vi "Init Actor Core.vi"(8 "error in (no error)":errorcluster, 11 "Monitor-Pulse in":refnum<class "Monitor-Pulse.lvclass">) -> (0 "error out":errorcluster, 3 "Monitor-Pulse out":refnum<class "Monitor-Pulse.lvclass">)   [LabVIEW 2015, in "Monitor-Pulse.lvclass"]
uses:
  Monitor-Pulse.lvclass
  Pulse Controller/Pulse Controller.lvclass
  Pulse Recorders/Red Pitaya Digitizer/Red Pitaya Digitizer.lvclass
  PulseEcho/PulsedFieldEcho/Pulse Echo Actor Project/Gage digitizer actor/Gage digitizer actor.lvclass
  <vilib>/ActorFramework/Actor/Actor.lvclass/Actor.ctl
  <vilib>/ActorFramework/Message Enqueuer/Message Enqueuer.lvclass/Message Enqueuer.ctl
  Measure Controller/Measure Controller.lvclass/Measure Controller.ctl
  <vilib>/ActorFramework/Message Enqueuer/Init from Existing Queue.vi
  <vilib>/ActorFramework/Message Enqueuer/Enqueue.vi
  <vilib>/ActorFramework/Message Priority Queue/Priority Enqueue.vi
  Measure Controller/Measure Controller.lvclass
  <vilib>/ActorFramework/Message Enqueuer/Message Enqueuer.lvclass
  Measure Object Messages/Open Front Panel Msg/Open Front Panel Msg.lvclass
  <vilib>/ActorFramework/Actor/Actor.lvclass
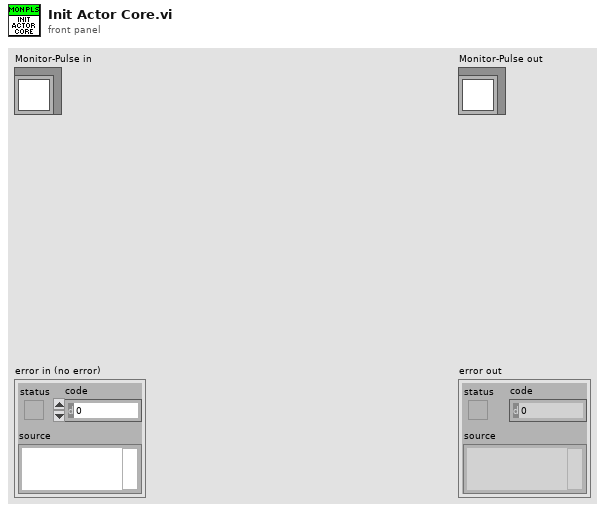
[diagram p1: front panel]
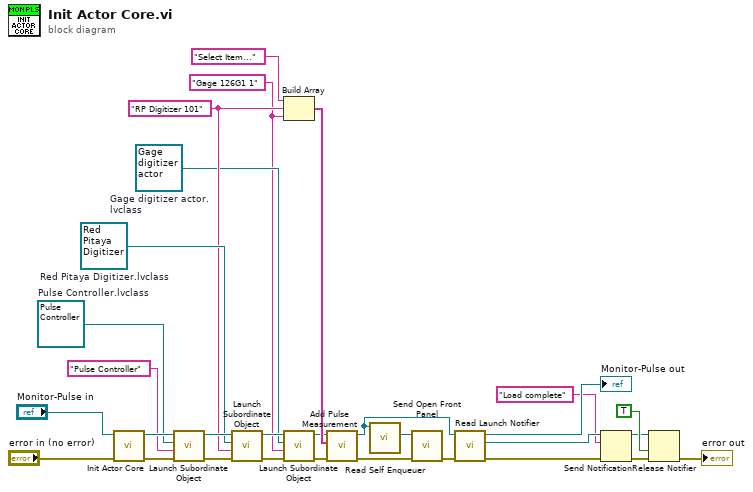
[diagram p0: block diagram]
diagram:
  w4 = refnum<class "Gage digitizer actor.lvclass"> refnum  # Gage digitizer actor.lvclass
  w3 = "Gage 126G1 1" ("Name")
  w13 = "RP Digitizer 101" ("Name")
  w16 = refnum<class "Red Pitaya Digitizer.lvclass"> refnum  # Red Pitaya Digitizer.lvclass
  w27 = refnum<class "Pulse Controller.lvclass"> refnum  # Pulse Controller.lvclass
  n1 = call-parent "Init Actor Core.vi"("error in (no error)"="error in (no error)", "Measure Object in"="Monitor-Pulse in") -> ("error out"=w25:errorcluster, "Measure Object out"=w28:refnum<class "Monitor-Pulse.lvclass">)  [unwired: 8 in]
  n2 = call-dynamic "Launch Subordinate Object.vi"("error in (no error)"=w25, "Name"="Pulse Controller", "Subordinate Object"=w27, "Measure Object in"=w28) -> ("error out"=w15:errorcluster, "Measure Object out"=w17:refnum<class "Monitor-Pulse.lvclass">)  [unwired: 5 in, 1 out]
  n3 = call-dynamic "Launch Subordinate Object.vi"("error in (no error)"=w15, "Name"=w13, "Subordinate Object"=w16, "Measure Object in"=w17) -> ("error out"=w5:errorcluster, "Measure Object out"=w6:refnum<class "Monitor-Pulse.lvclass">)  [unwired: 5 in, 1 out]
  n4 = Build Array("Select Item..." ("element"), w13, w3) -> (w8:string[])
  n5 = call-dynamic "Launch Subordinate Object.vi"("error in (no error)"=w5, "Name"=w3, "Subordinate Object"=w4, "Measure Object in"=w6) -> ("error out"=w2:errorcluster, "Measure Object out"=w1:refnum<class "Monitor-Pulse.lvclass">)  [unwired: 5 in, 1 out]
  n6 = call-dynamic "Add Pulse Measurement.vi"("error in (no error)"=w2, "Item Names"=w8, "Monitor-Pulse in"=w1) -> ("error out"=w12:errorcluster, "Monitor-Pulse out"=w14:refnum<class "Monitor-Pulse.lvclass">)  [unwired: 7 in]
  n7 = call <vilib>:"Read Self Enqueuer.vi"("Actor"=w14) -> ("Self Enqueuer"=w24:refnum<class "Message Enqueuer.lvclass">)  [unwired: 10 in]
  n8 = call "Send Open Front Panel.vi"("error in (no error)"=w12, "Message Enqueuer"=w24) -> ("error out"=w11:errorcluster)  [unwired: 8 in, 1 out]
  n9 = call "Read Launch Notifier.vi"("error in (no error)"=w11, "Measure Controller in"=w14) -> ("error out"=w10:errorcluster, "Launch Notifier"=w20:refnum<notifier>, "Measure Controller out"=→"Monitor-Pulse out":refnum<class "Monitor-Pulse.lvclass">)  [unwired: 7 in]
  n10 = Send Notification(notification="Load complete" ("Message"), notifier=w20, error in (no error)=w10) -> (notifier out=w19:refnum<notifier>, error out=w21:errorcluster)
  n11 = Release Notifier(notifier=w19, force destroy? (F)=TRUE ("Kill notifier"), error in (no error)=w21) -> (error out=→"error out":errorcluster)  [unwired: 2 out]
